vi "Write ID.vi"(8 "error in (no error)":errorcluster, 10 "id":string, 11 "SVGImage in":refnum<class "SVGImage.lvclass">) -> (0 "error out":errorcluster, 3 "SVGImage out":refnum<class "SVGImage.lvclass">)   [LabVIEW 2019, in "SVGImage.lvclass"]
uses:
  SVGImage.lvclass
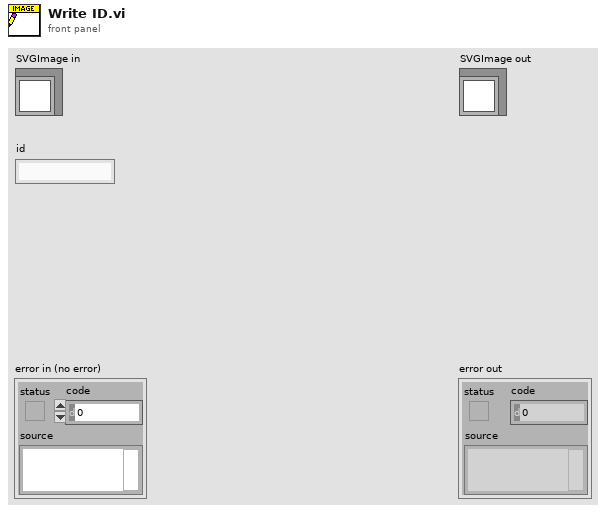
[diagram p1: front panel]
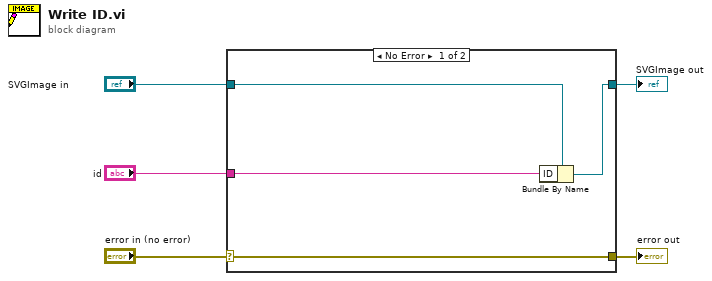
[diagram p0: block diagram]
diagram:
  n1 = case shown="No Error" "error in (no error)" {
    selector: "error in (no error)" -> [w9 w10]
    tunnel: [w9 w10] -> w4
    tunnel: [w7 w11] -> w2
    tunnel: "SVGImage in" -> [w8 w11]
    tunnel: "id" -> [w6 _]
    frame No Error {
      n2 = Bundle By Name(cluster=w8, "ID"=w6) -> (w7:refnum<class "SVGImage.lvclass">)
    }
    frame Error {
    }
  }
  "error out" <- w4
  "SVGImage out" <- w2
